vi "Interpret Driver Controls.vi"   [LabVIEW 2018]
uses:
  SubSystems/Controllers/Driver Controller/Driver Controller Global.vi
  SubSystems/Drive Train/Drive Train Global.vi
  SubSystems/Lift/Lift Global.vi
  SubSystems/Controllers/Manipulator Controlller/Manipulator Controller Global.vi
  SubSystems/Cargo Intake/Cargo Intake Global.vi
  SubSystems/Hatch Panel Intake/Hatch Panel Intake Global.vi
types:
  T1 = cluster{"Rollover":dbl, "Yaw":dbl, "Cont Yaw":dbl}
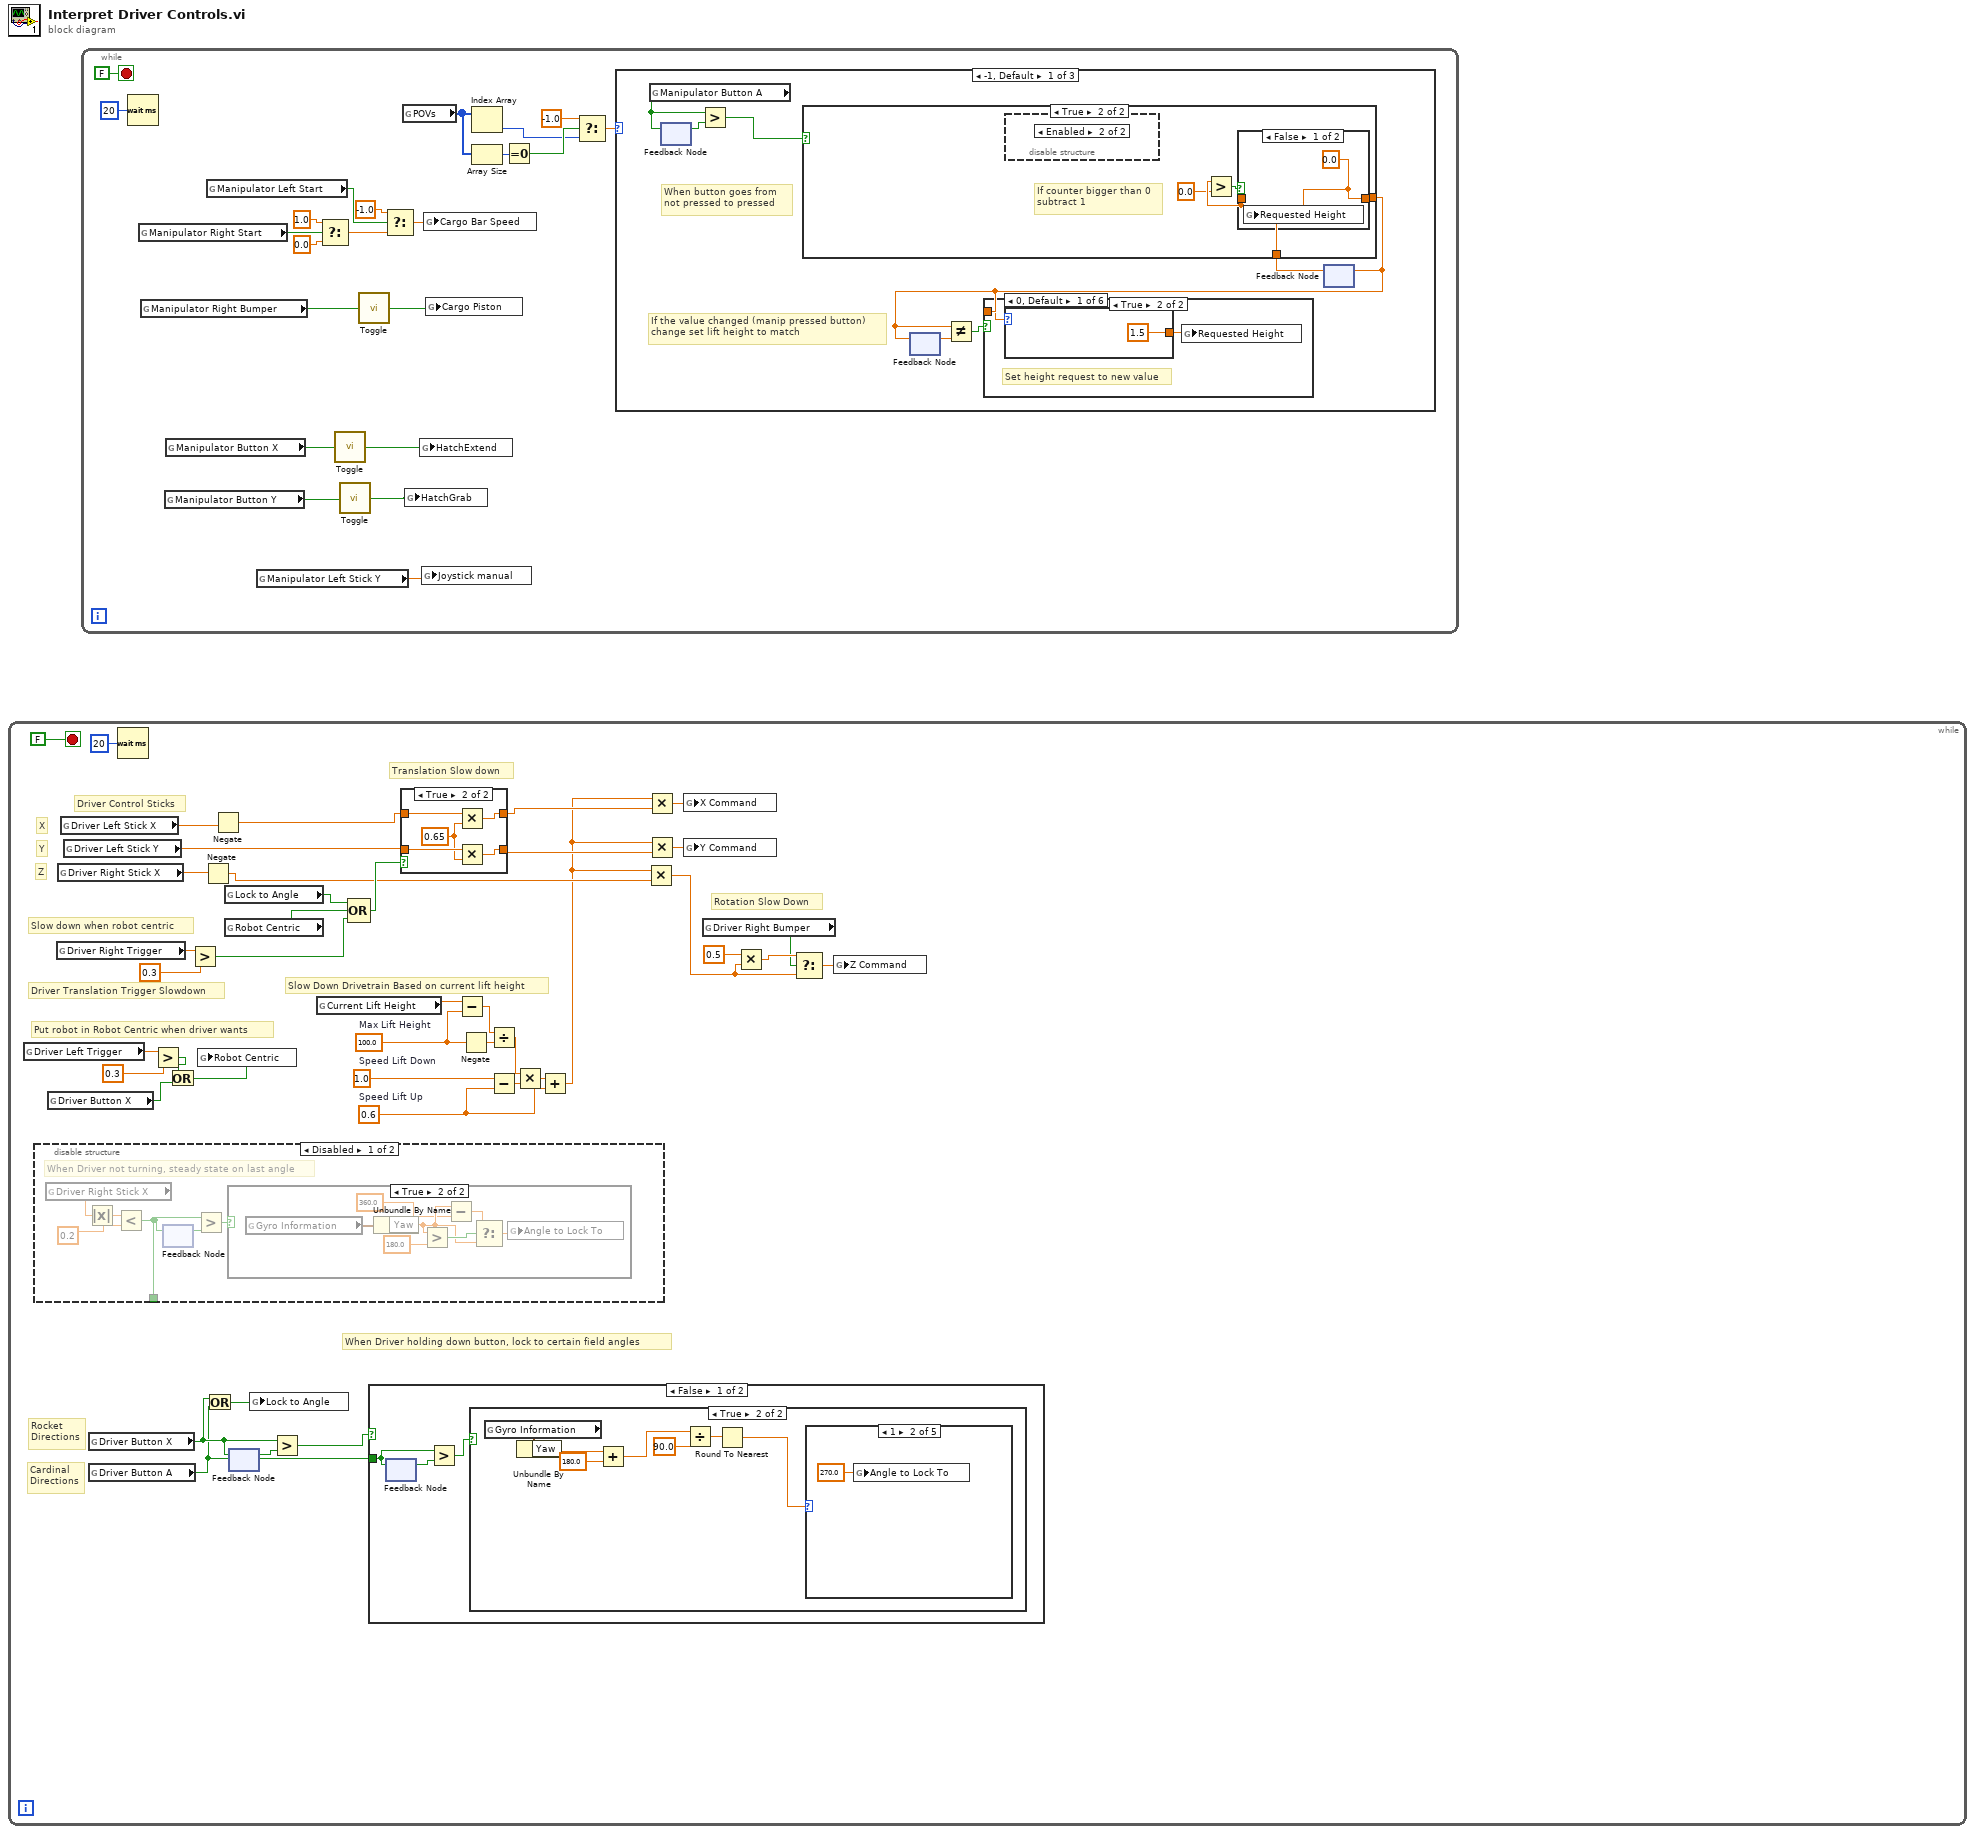
[diagram p0: block diagram]
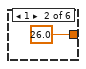
[diagram p3: hidden frame]
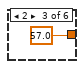
[diagram p4: hidden frame]
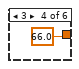
[diagram p5: hidden frame]
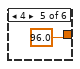
[diagram p6: hidden frame]
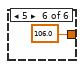
[diagram p7: hidden frame]
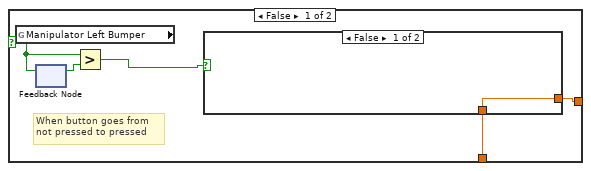
[diagram p8: hidden frame]
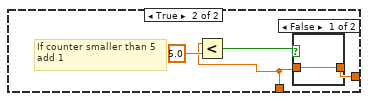
[diagram p9: hidden frame]
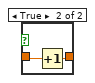
[diagram p10: hidden frame]
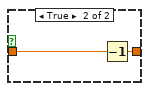
[diagram p11: hidden frame]
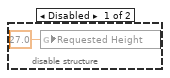
[diagram p12: hidden frame]
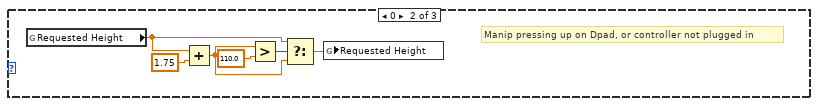
[diagram p13: hidden frame]
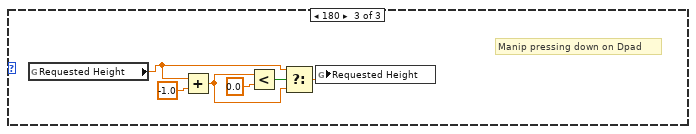
[diagram p14: hidden frame]
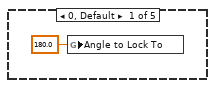
[diagram p18: hidden frame]
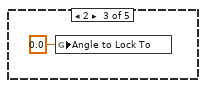
[diagram p19: hidden frame]
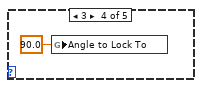
[diagram p20: hidden frame]
diagram:
  n1 = while {
    stop <- FALSE stop-if-true
    w13 = 0.6  # Speed Lift Up
    w17 = 1.0  # Speed Lift Down
    w11 = 100.0  # Max Lift Height
    # "Rotation Slow Down"
    # "Rocket\nDirections"
    # "Cardinal\nDirections"
    # "When Driver holding down button, lock to certain field angles"
    # "Slow Down Drivetrain Based on current lift height"
    # "Put robot in Robot Centric when driver wants"
    # "Slow down when robot centric"
    # "Driver Translation Trigger Slowdown"
    # "Translation Slow down"
    # "Z"
    # "Y"
    # "X"
    # "Driver Control Sticks"
    n2 = global read "Driver Controller Global.vi" "Driver Left Trigger"() -> (w33:dbl)
    n3 = disable-structure shown="Disabled" {
      disable-tunnel: [w43 _] -> _
      frame Disabled {
        # "When Driver not turning, steady state on last angle"
        n4 = global read "Driver Controller Global.vi" "Driver Right Stick X"() -> (w44:dbl)
        n5 = Absolute Value(x=w44) -> (abs(x)=w48:dbl)
        n6 = Less?(x=w48, y=0.2) -> (x < y?=w43:bool)
        n7 = feedback #1() -> (w46:bool)  [unwired: 1 in]
        n8 = feedback-in #1(w43) -> ()
        n9 = Greater?(x=w43, y=w46) -> (0:w45:bool)
        n10 = case shown="True" w45 {
          frame False {
          }
          frame True {
            n11 = global read "Drive Train Global.vi" "Gyro Information"() -> (w55:T1)
            n12 = Unbundle By Name(w55) -> ("Yaw"=w52:dbl)
            n13 = Greater?(x=w52, y=180.0) -> (0:w53:bool)
            n14 = Subtract(x=w52, y=360.0) -> (x-y=w50:dbl)
            n15 = Select(t=w50, s=w53, f=w52) -> (s? t:f=w49:dbl)
            n16 = global write "Drive Train Global.vi" "Angle to Lock To"(w49) -> ()
          }
        }
      }
      frame Enabled {
      }
    }
    n17 = global read "Driver Controller Global.vi" "Driver Button X"() -> (w2:bool)
    n18 = global read "Driver Controller Global.vi" "Driver Right Trigger"() -> (w38:dbl)
    n19 = global read "Driver Controller Global.vi" "Driver Right Stick X"() -> (w39:dbl)
    n20 = global read "Driver Controller Global.vi" "Driver Left Stick X"() -> (w40:dbl)
    n21 = global read "Driver Controller Global.vi" "Driver Left Stick Y"() -> (w20:dbl)
    n22 = global read "Driver Controller Global.vi" "Driver Button X"() -> (w8:bool)
    n23 = global read "Driver Controller Global.vi" "Driver Button A"() -> (w6:bool)
    n24 = Wait (ms)(milliseconds to wait=u32 20) -> ()  [unwired: 1 out]
    n25 = Greater?(x=w33, y=0.3) -> (0:w4:bool)
    n26 = Or(x=w4, y=w2) -> (x .or. y?=w3:bool)
    n27 = Greater?(x=w38, y=0.3) -> (0:w28:bool)
    n28 = global write "Drive Train Global.vi" "Robot Centric"(w3) -> ()
    n29 = Negate(x=w39) -> (-x=w24:dbl)
    n30 = Or(x=w8, y=w6) -> (x .or. y?=w5:bool)
    n31 = Negate(x=w40) -> (-x=w21:dbl)
    n32 = global read "Drive Train Global.vi" "Lock to Angle"() -> (w1:bool)
    n33 = global read "Drive Train Global.vi" "Robot Centric"() -> (w27:bool)
    n34 = feedback #2() -> (w9:bool)  [unwired: 1 in]
    n35 = feedback-in #2(w8) -> ()
    n36 = global write "Drive Train Global.vi" "Lock to Angle"(w5) -> ()
    n37 = Greater?(x=w8, y=w9) -> (0:w7:bool)
    n38 = global read "Lift Global.vi" "Current Lift Height"() -> (w19:dbl)
    n39 = Compound Arithmetic op=OR(w1, w27, w28) -> (w26:bool)
    n40 = case shown="False" w7 {
      tunnel: w6 -> [w57 _]
      frame False {
        n41 = feedback #3() -> (w58:bool)  [unwired: 1 in]
        n42 = feedback-in #3(w57) -> ()
        n43 = Greater?(x=w57, y=w58) -> (0:w56:bool)
        n44 = case shown="True" w56 {
          frame False {
          }
          frame True {
            n45 = global read "Drive Train Global.vi" "Gyro Information"() -> (w65:T1)
            n46 = Unbundle By Name(w65) -> ("Yaw"=w62:dbl)
            n47 = Add(x=w62, y=180.0) -> (x+y=w61:dbl)
            n48 = Divide(x=w61, y=90.0) -> (x/y=w63:dbl)
            n49 = Round To Nearest(number=w63) -> (nearest integer value=w59:dbl)
            n50 = case shown="1" w59 {
              frame 0, Default {
                n51 = global write "Drive Train Global.vi" "Angle to Lock To"(180.0 ("Angle to Lock To")) -> ()
              }
              frame 1 {
                n52 = global write "Drive Train Global.vi" "Angle to Lock To"(270.0 ("Angle to Lock To")) -> ()
              }
              frame 2 {
                n53 = global write "Drive Train Global.vi" "Angle to Lock To"(0.0 ("Angle to Lock To")) -> ()
              }
              frame 3 {
                n54 = global write "Drive Train Global.vi" "Angle to Lock To"(90.0 ("Angle to Lock To")) -> ()
              }
              frame 4 {
                n55 = global write "Drive Train Global.vi" "Angle to Lock To"(180.0 ("Angle to Lock To")) -> ()
              }
            }
          }
        }
      }
      frame True {
        n56 = global read "Drive Train Global.vi" "Gyro Information"() -> (w79:T1)
        n57 = Unbundle By Name(w79) -> ("Cont Yaw"=w77:dbl)
        n58 = Quotient & Remainder(x=w77, y=360.0) -> (x-y*floor(x/y)=w75:dbl)  [unwired: 1 out]
        n59 = Divide(x=w75, y=60.0) -> (x/y=w71:dbl)
        n60 = In Range and Coerce(upper limit=1.5, x=w71, lower limit=0.0) -> (In Range?=w72:bool)  [unwired: 1 out]
        n61 = case shown="False" w72 {
          tunnel: w71 -> [w80 _]
          frame False {
            n62 = In Range and Coerce(upper limit=3.0, x=w80, lower limit=1.5) -> (In Range?=w81:bool)  [unwired: 1 out]
            n63 = case shown="False" w81 {
              tunnel: w80 -> [w86 _]
              tunnel: w80 -> [w84 _]
              frame False {
                n64 = In Range and Coerce(upper limit=4.5, x=w86, lower limit=3.0) -> (In Range?=w85:bool)  [unwired: 1 out]
                n65 = case shown="False" w85 {
                  tunnel: w84 -> [w90 _]
                  frame False {
                    n66 = In Range and Coerce(upper limit=6.0, x=w90, lower limit=4.5) -> (In Range?=w89:bool)  [unwired: 1 out]
                    n67 = case shown="True" w89 {
                      frame False {
                      }
                      frame True {
                        n68 = global write "Drive Train Global.vi" "Angle to Lock To"(330.0 ("Angle to Lock To")) -> ()
                      }
                    }
                  }
                  frame True {
                    n69 = global write "Drive Train Global.vi" "Angle to Lock To"(210.0 ("Angle to Lock To")) -> ()
                  }
                }
              }
              frame True {
                n70 = global write "Drive Train Global.vi" "Angle to Lock To"(150.0 ("Angle to Lock To")) -> ()
              }
            }
          }
          frame True {
            n71 = global write "Drive Train Global.vi" "Angle to Lock To"(30.0 ("Angle to Lock To")) -> ()
          }
        }
      }
    }
    n72 = case shown="True" w26 {
      tunnel: w20 -> [w98 w103]
      tunnel: [w98 w102] -> w23
      tunnel: [w97 w101] -> w22
      tunnel: w21 -> [w97 w100]
      frame False {
      }
      frame True {
        w99 = 0.65 ("Y Slower")
        n73 = Multiply(x=w100, y=w99) -> (x*y=w101:dbl)
        n74 = Multiply(x=w103, y=w99) -> (x*y=w102:dbl)
      }
    }
    n75 = Subtract(x=w19, y=w11) -> (x-y=w18:dbl)
    n76 = Negate(x=w11) -> (-x=w12:dbl)
    n77 = Divide(x=w18, y=w12) -> (x/y=w16:dbl)
    n78 = Subtract(x=w17, y=w13) -> (x-y=w15:dbl)
    n79 = Multiply(x=w16, y=w15) -> (x*y=w14:dbl)
    n80 = Add(x=w14, y=w13) -> (x+y=w10:dbl)
    n81 = Multiply(x=w10, y=w24) -> (x*y=w32:dbl)
    n82 = Multiply(x=w10, y=w22) -> (x*y=w36:dbl)
    n83 = Multiply(x=w10, y=w23) -> (x*y=w35:dbl)
    n84 = global write "Drive Train Global.vi" "X Command"(w36) -> ()
    n85 = global write "Drive Train Global.vi" "Y Command"(w35) -> ()
    n86 = global read "Driver Controller Global.vi" "Driver Right Bumper"() -> (w29:bool)
    n87 = Multiply(x=0.5, y=w32) -> (x*y=w31:dbl)
    n88 = Select(t=w31, s=w29, f=w32) -> (s? t:f=w25:dbl)
    n89 = global write "Drive Train Global.vi" "Z Command"(w25) -> ()
  }
  n90 = while {
    stop <- FALSE stop-if-true
    n91 = Wait (ms)(milliseconds to wait=u32 20) -> ()  [unwired: 1 out]
    n92 = global read "Manipulator Controller Global.vi" "Manipulator Right Start"() -> (w120:bool)
    n93 = global read "Manipulator Controller Global.vi" "Manipulator Right Bumper"() -> (w123:bool)
    n94 = global read "Manipulator Controller Global.vi" "Manipulator Button Y"() -> (w114:bool)
    n95 = global read "Manipulator Controller Global.vi" "Manipulator Button X"() -> (w112:bool)
    n96 = global read "Manipulator Controller Global.vi" "Manipulator Left Start"() -> (w119:bool)
    n97 = global read "Manipulator Controller Global.vi" "Manipulator Left Stick Y"() -> (w104:dbl)
    n98 = Select(t=1.0, s=w120, f=0.0) -> (s? t:f=w118:dbl)
    n99 = call "Toggle.vi"("Input"=w112) -> ("Output"=w113:bool)
    n100 = call "Toggle.vi"("Input"=w114) -> ("Output"=w105:bool)
    n101 = call "Toggle.vi"("Input"=w123) -> ("Output"=w122:bool)
    n102 = Select(t=-1.0, s=w119, f=w118) -> (s? t:f=w121:dbl)
    n103 = global read "Manipulator Controller Global.vi" "POVs"() -> (w111:i16[])
    n104 = global write "Hatch Panel Intake Global.vi" "HatchGrab"(w105) -> ()
    n105 = global write "Hatch Panel Intake Global.vi" "HatchExtend"(w113) -> ()
    n106 = global write "Lift Global.vi" "Joystick manual"(w104) -> ()
    n107 = global write "Cargo Intake Global.vi" "Cargo Bar Speed"(w121) -> ()
    n108 = global write "Cargo Intake Global.vi" "Cargo Piston"(w122) -> ()
    n109 = Index Array(array=w111) -> (element=w106:i16)  [unwired: 1 in]
    n110 = Array Size(array=w111) -> (size(s)=w110:i32)
    n111 = Equal To 0?(x=w110) -> (x = 0?=w108:bool)
    n112 = Select(t=-1.0, s=w108, f=w106) -> (s? t:f=w109:dbl)
    n113 = case shown="-1, Default" w109 {
      frame -1, Default {
        # "If the value changed (manip pressed button)\nchange set lift height to match"
        # "When button goes from\nnot pressed to pressed"
        n114 = global read "Manipulator Controller Global.vi" "Manipulator Button A"() -> (w131:bool)
        n115 = feedback #4() -> (w132:bool)  [unwired: 1 in]
        n116 = feedback-in #4(w131) -> ()
        n117 = Greater?(x=w131, y=w132) -> (0:w126:bool)
        n118 = feedback #5() -> (w129:dbl)  [unwired: 1 in]
        n119 = feedback #6() -> (w130:dbl)  [unwired: 1 in]
        n120 = case shown="True" w126 {
          tunnel: [w142 w157] -> w128
          tunnel: w130 -> [w143 w156]
          frame False {
            # "When button goes from\nnot pressed to pressed"
            n121 = global read "Manipulator Controller Global.vi" "Manipulator Left Bumper"() -> (w145:bool)
            n122 = feedback #7() -> (w144:bool)  [unwired: 1 in]
            n123 = feedback-in #7(w145) -> ()
            n124 = Greater?(x=w145, y=w144) -> (0:w141:bool)
            n125 = case shown="False" w141 {
              tunnel: w143 -> [w146 w148]
              tunnel: [w146 w150] -> w142
              frame False {
              }
              frame True {
                # "If counter smaller than 5\nadd 1"
                n126 = Less?(x=w148, y=5.0) -> (x < y?=w147:bool)
                n127 = case shown="False" w147 {
                  tunnel: [w151 w153] -> w150
                  tunnel: w148 -> [w151 w152]
                  frame False {
                  }
                  frame True {
                    n128 = Increment(x=w152) -> (x+1=w153:dbl)
                  }
                }
              }
            }
          }
          frame True {
            # "If counter bigger than 0\nsubtract 1"
            n129 = disable-structure shown="Enabled" {
              frame Disabled {
                n130 = global write "Lift Global.vi" "Requested Height"(27.0 ("Requested Height")) -> ()
              }
              frame Enabled {
              }
            }
            n131 = Greater?(x=w156, y=0.0) -> (0:w155:bool)
            n132 = case shown="False" w155 {
              tunnel: [w158 w160] -> w157
              tunnel: w156 -> [_ w159]
              frame False {
                w158 = 0.0 ("y")
                n133 = global write "Lift Global.vi" "Requested Height"(w158) -> ()
              }
              frame True {
                n134 = Decrement(x=w159) -> (x-1=w160:dbl)
              }
            }
          }
        }
        n135 = feedback-in #5(w128) -> ()
        n136 = Not Equal?(x=w128, y=w129) -> (x != y?=w127:bool)
        n137 = case shown="True" w127 {
          tunnel: w128 -> [_ w133]
          frame False {
            # "Manipulator didnt request change"
          }
          frame True {
            # "Set height request to new value"
            n138 = case shown="0, Default" w133 {
              tunnel: [1.5 ("Requested Height") 26.0 ("Requested Height") 57.0 ("Requested Height") 66.0 ("Requested Height") 96.0 ("Requested Height") 106.0 ("Requested Height")] -> w134
              frame 0, Default {
              }
              frame 1 {
              }
              frame 2 {
              }
              frame 3 {
              }
              frame 4 {
              }
              frame 5 {
              }
            }
            n139 = global write "Lift Global.vi" "Requested Height"(w134) -> ()
          }
        }
        n140 = feedback-in #6(w128) -> ()
      }
      frame 0 {
        # "Manip pressing up on Dpad, or controller not plugged in"
        n141 = global read "Lift Global.vi" "Requested Height"() -> (w163:dbl)
        n142 = Add(x=w163, y=1.75) -> (x+y=w162:dbl)
        n143 = Greater?(x=w162, y=110.0) -> (0:w164:bool)
        n144 = Select(t=w163, s=w164, f=w162) -> (s? t:f=w165:dbl)
        n145 = global write "Lift Global.vi" "Requested Height"(w165) -> ()
      }
      frame 180 {
        # "Manip pressing down on Dpad"
        n146 = global read "Lift Global.vi" "Requested Height"() -> (w168:dbl)
        n147 = Add(x=w168, y=-1.0) -> (x+y=w170:dbl)
        n148 = Less?(x=w170, y=0.0) -> (x < y?=w171:bool)
        n149 = Select(t=w168, s=w171, f=w170) -> (s? t:f=w169:dbl)
        n150 = global write "Lift Global.vi" "Requested Height"(w169) -> ()
      }
    }
  }
